vi "CDEx PID Design with Dimensionless Alpha.vi"() -> ()   [LabVIEW 2020]
doc: "This example demonstrates how changing the topology of a PID controller can give completely different results even if you use the same coefficients. This examples shows that you must know the topology of the controller before obtaining the coefficients."
uses:
  <vilib>/addons/Control Design/_Model Construction/Data Typedefs.llb/CD Time Info.ctl
  <vilib>/addons/Control Design/_Model Construction/NI_LinSys_Data Typedefs.lvlib
  <vilib>/addons/Control Design/_Dynamic Analysis/NI_CD_Dynamic Analysis.lvlib
  <vilib>/addons/Control Design/_Dynamic Analysis/Dynamic Analysis.llb/Dynamic Analysis subVI/cd_Pole-Zero Map (Transfer Function).vi
  <vilib>/addons/Control Design/_Model Construction/NI_LinSys_Model Creation.lvlib
  <vilib>/addons/Control Design/_Model Construction/Model Creation.llb/Model Creation SubVI/cd_Create Transfer Function Model.vi
  <vilib>/addons/Control Design/_Time Response Analysis/NI_CD_Time Response.lvlib
  <vilib>/addons/Control Design/_Time Response Analysis/Time Response.llb/Time Response subVI/cd_Step Response (Transfer Function).vi
  <vilib>/addons/Control Design/_Model Interconnection/NI_CD_Model Interconnection.lvlib
  <vilib>/addons/Control Design/_Model Interconnection/Model Interconnection.llb/Model Interconnection SubVI/cd_Feedback (TF and TF).vi
  <vilib>/addons/Control Design/_Utility/NI_CD_Model Viewer.lvlib
  <vilib>/addons/Control Design/_Utility/Model Viewer.llb/Model Viewer SubVI/cd_Draw Zero-Pole-Gain Equation (TF).vi
  <vilib>/addons/Control Design/_Model Construction/NI_CD_Special Model Creation.lvlib
  <vilib>/addons/Control Design/_Model Construction/Special Model Creation.llb/Special Model Creation SubVI/CD Create PID Academic Model.vi
  <vilib>/addons/Control Design/_Model Construction/Special Model Creation.llb/Special Model Creation SubVI/CD Create PID Parallel Model.vi
  <vilib>/addons/Control Design/_Model Construction/Special Model Creation.llb/Special Model Creation SubVI/CD Create PID Series Model.vi
  <vilib>/addons/Control Design/_Model Interconnection/Model Interconnection.llb/Model Interconnection SubVI/cd_Series (TF and TF).vi
panel:
  in  "Plant Type":u16(ring) items=["One Pole", "Two Real Poles", "One Pole with Integrator", "Complex Poles", "Two Complex with Integrator", "Two Integrators"]
  out "Plant":picture
  out "PID Controller":picture
  out "Control Effort [y(s)/u(s)]":cluster{"time":dbl[], dbl[]}[](graph)
  in  "PID Topology":u16(ring) items=["PID Academic", "PID Parallel", "PID Series"]
  in  "stop":bool
  out "Reference Tracking [y(s)/r(s)]":cluster{"time":dbl[], dbl[]}[](graph)
  out "Pole-Zero Map":cluster{dbl[], dbl[]}[](graph)
  in  "Alpha":dbl(slide) scale=0.0..1.0
  in  "Derivative Coefficient":dbl(slide) scale=0.0..10.0
  in  "Integral Coefficient":dbl(slide)=0.10204081632653061 scale=0.0..10.0
  in  "Proportional Gain (Kc)":dbl(slide)=1.0204081632653061 scale=0.0..20.0
  # "d(s)"
  # "+"
  # "r(s)"
  # "y(s)"
  # "+"
  # "+"
  # "u(s)"
  # "-"
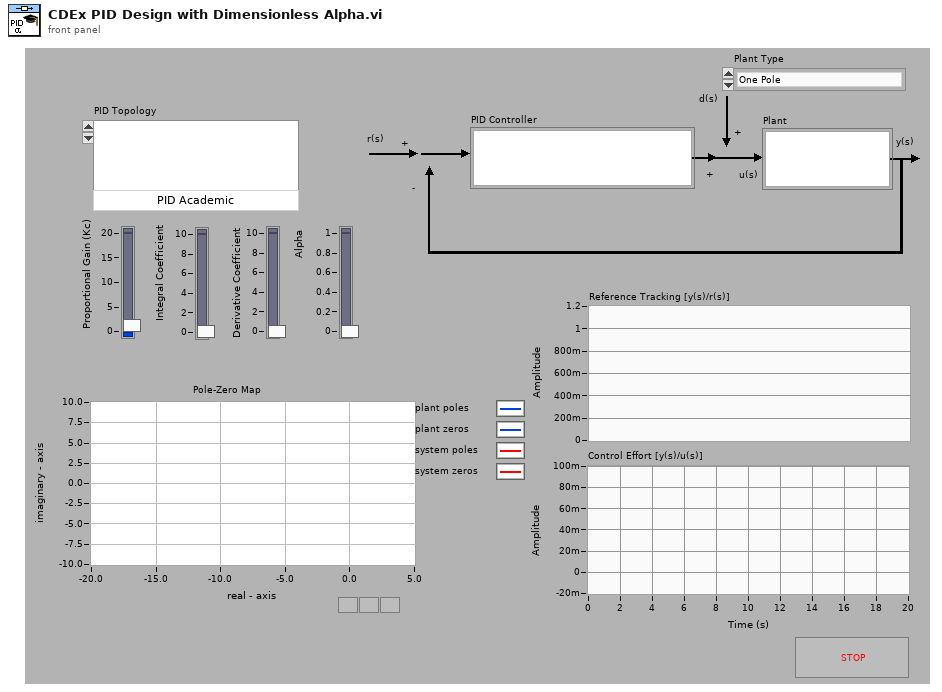
[diagram p1: front panel]
types:
  T1 = typedef "NI_LinSys_Data Typedefs.lvlib/CD Time Info.ctl" = cluster{"t0":dbl, "dt":dbl, "tf":dbl}
  T2 = typedef "NI_LinSys_Model Typedefs.lvlib/CD Transfer Function Model (MIMO).ctl" = cluster{"properties":T3, "transfer function(s)":T4[][]}
  T3 = typedef "NI_LinSys_Model Typedefs.lvlib/CD General Elements.ctl" = cluster{"Model name":string, "Input names":string[], "Output names":string[], "Input Delays":dbl[], "Output Delays":dbl[], "Sampling Time":dbl, "Notes":string}
  T4 = typedef "NI_LinSys_Model Typedefs.lvlib/CD Transfer Function Model (SISO).ctl" = cluster{"Numerator":dbl[], "Denominator":dbl[], "delay":dbl}
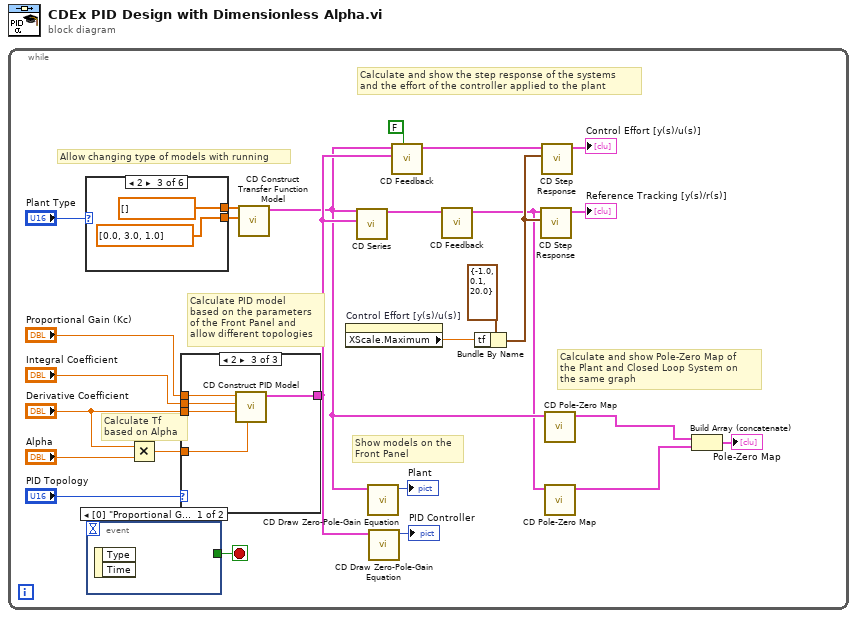
[diagram p0: block diagram]
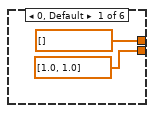
[diagram p2: hidden frame]
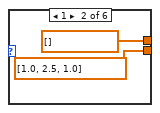
[diagram p3: hidden frame]
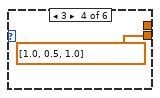
[diagram p4: hidden frame]
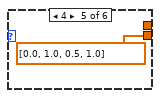
[diagram p5: hidden frame]
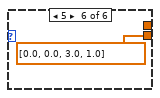
[diagram p6: hidden frame]
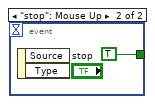
[diagram p7: hidden frame]
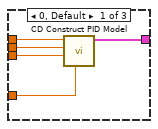
[diagram p8: hidden frame]
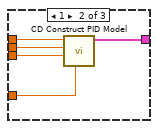
[diagram p9: hidden frame]
diagram:
  n1 = while {
    stop <- w16 stop-if-true
    # "Calculate and show the step response of the systems\nand the effort of the controller applied to the plant"
    # "Calculate and show Pole-Zero Map of \nthe Plant and Closed Loop System on\nthe same graph"
    # "Show models on the\nFront Panel"
    # "Calculate Tf\nbased on Alpha"
    # "Calculate PID model\nbased on the parameters\nof the Front Panel and\nallow different topologies"
    # "Allow changing type of models with running"
    n2 = case shown="2" "Plant Type" {
      tunnel: [dbl[] [1.0, 1.0] ("Denominator") dbl[] [1.0, 2.5, 1.0] ("Denominator") dbl[] [0.0, 3.0, 1.0] ("Denominator") dbl[] [1.0, 0.5, 1.0] ("Denominator") dbl[] [0.0, 1.0, 0.5, 1.0] ("Denominator") dbl[] [0.0, 0.0, 3.0, 1.0] ("Denominator")] -> w7
      tunnel: [dbl[] [] ("Denominator") dbl[] [] ("Denominator") dbl[] [] ("Denominator") _ _ _] -> w6
      frame 0, Default {
      }
      frame 1 {
      }
      frame 2 {
      }
      frame 3 {
      }
      frame 4 {
      }
      frame 5 {
      }
    }
    n3 = event shown="[0] \"Proportional Gain (Kc)\", \"Integral Coefficient\", \"Derivative Coefficient\", \"Alpha\", \"PID Topology\", \"Plant Type\": Value Change;  \"Reference Tracking [y(s)/r(s)]\", \"Control Effort [y(s)/u(s)]\": Scale Range Change" {
      selector: _ -> [_ _]
      dyn-events: _ -> [_ _]
      timeout: _ -> [_ _]
      tunnel: [_ TRUE] -> w16
      event "Proportional Gain (Kc)", "Integral Coefficient", "Derivative Coefficient", "Alpha", "PID Topology", "Plant Type": Value Change; "Reference Tracking [y(s)/r(s)]", "Control Effort [y(s)/u(s)]": Scale Range Change {
        n4 = event-data() -> ()  [unwired: 1 in, 2 out]
      }
      event "stop": Mouse Up {
        n5 = event-data() -> ()  [unwired: 1 in, 2 out]
      }
    }
    n6 = Multiply(x="Derivative Coefficient", y="Alpha") -> (x*y=w23:dbl)
    n7 = case shown="2" "PID Topology" {
      tunnel: "Proportional Gain (Kc)" -> [w41 w46 w51]
      tunnel: "Integral Coefficient" -> [w40 w45 w50]
      tunnel: "Derivative Coefficient" -> [w37 w42 w47]
      tunnel: w23 -> [w39 w44 w49]
      tunnel: [w38 w43 w48] -> w11
      frame 0, Default {
        n8 = call-poly <vilib>:"CD Construct PID Model.vi"("High Frequency Time Constant [s] (Tf)"=w39, "Derivative time [s] (Td)"=w37, "Integral time [s] (Ti)"=w40, "Proportional Gain (Kc)"=w41) -> ("Transfer Function Model"=w38:T2)  [unwired: 6 in, 1 out]
      }
      frame 1 {
        n9 = call-poly <vilib>:"CD Construct PID Model.vi"("High Frequency Time Constant [s] (Tf)"=w44, "Derivative Gain (Kd)"=w42, "Integral Gain (Ki)"=w45, "Proportional Gain (Kp)"=w46) -> ("Transfer Function Model"=w43:T2)  [unwired: 6 in, 1 out]
      }
      frame 2 {
        n10 = call-poly <vilib>:"CD Construct PID Model.vi"("High Frequency Time Constant [s] (Tf)"=w49, "Derivative Time [s] (TD)"=w47, "Integral Time [s] (TI)"=w50, "Proportional Gain (KC)"=w51) -> ("Transfer Function Model"=w48:T2)  [unwired: 6 in, 1 out]
      }
    }
    n11 = call-poly <vilib>:"CD Construct Transfer Function Model.vi"("Denominator"=w7, "Numerator"=w6) -> ("Transfer Function Model"=w4:T2)  [unwired: 8 in, 1 out]
    n12 = property on="Control Effort [y(s)/u(s)]" class="XYGraph (strict)"() -> ("XScale.Maximum"=w9:dbl)  [unwired: 2 in, 2 out]
    n13 = call-poly <vilib>:"CD Series.vi"("Model 2"=w11, "Model 1"=w4) -> ("Series Model"=w20:T2)  [unwired: 8 in, 1 out]
    n14 = call-poly <vilib>:"CD Draw Zero-Pole-Gain Equation.vi"("Transfer Function Model"=w4) -> ("Equation"=→"Plant":picture)  [unwired: 8 in, 2 out]
    n15 = call-poly <vilib>:"CD Draw Zero-Pole-Gain Equation.vi"("Transfer Function Model"=w11) -> ("Equation"=→"PID Controller":picture)  [unwired: 8 in, 2 out]
    n16 = call-poly <vilib>:"CD Feedback.vi"("Feedback Sign"=FALSE, "Model 2"=w11, "Model 1"=w4) -> ("Closed-Loop Model"=w14:T2)  [unwired: 7 in, 1 out]
    n17 = call-poly <vilib>:"CD Feedback.vi"("Model 1"=w20) -> ("Closed-Loop Model"=w3:T2)  [unwired: 9 in, 1 out]
    n18 = Bundle By Name(cluster=T1 {"t0"=-1.0, "dt"=0.1, "tf"=20.0} ("Time Info"), "tf"=w9) -> (w10:T1)
    n19 = call-poly <vilib>:"CD Step Response.vi"("Time Range"=w10, "Transfer Function Model"=w3) -> ("Step Response Graph"=→"Reference Tracking [y(s)/r(s)]":cluster{"time":dbl[], dbl[]}[])  [unwired: 7 in, 2 out]
    n20 = call-poly <vilib>:"CD Step Response.vi"("Time Range"=w10, "Transfer Function Model"=w14) -> ("Step Response Graph"=→"Control Effort [y(s)/u(s)]":cluster{"time":dbl[], dbl[]}[])  [unwired: 7 in, 2 out]
    n21 = call-poly <vilib>:"CD Pole-Zero Map.vi"("Transfer Function Model"=w4) -> ("Pole-Zero Map"=w1:cluster{dbl[], dbl[]}[])  [unwired: 7 in, 3 out]
    n22 = call-poly <vilib>:"CD Pole-Zero Map.vi"("Transfer Function Model"=w3) -> ("Pole-Zero Map"=w5:cluster{dbl[], dbl[]}[])  [unwired: 7 in, 3 out]
    n23 = Build Array (concatenate)(w1, w5) -> (→"Pole-Zero Map":cluster{dbl[], dbl[]}[])
  }
